vi "Decimator.vi"(4 "Size":u32=10, 6 "Mode":T1(ring)=enum."Non-sliding block", 8 "error in (no error)":errorcluster, 9 "Reset":bool, 10 "Enable":bool=TRUE, 11 "Signals":dynamicdata(graph)) -> (0 "error out":errorcluster, 1 "Data Valid":bool, 3 "Mean":dynamicdata(graph), 5 "Maximum":dynamicdata(graph))   [LabVIEW 2014]
doc: "Acquires a large number of data points and compresses the data points into a smaller number of points.\n--------------------\n\nThis Express VI is configured as follows:\n\nReduction Factor: 10\nReduction Method: Maximum\nReduction Method: Mean"
panel:
  in  "Tab Control":T2(tab)
  out "Sum":dynamicdata(graph)
  out "Median":dynamicdata(graph)
  out "Minimum":dynamicdata(graph)
  out "Last":dynamicdata(graph)
  out "Waveform Output":dynamicdata(graph)
  out "Signals In":dynamicdata(graph)
  in  "Functions":bool[](array[boolean])=[FALSE, TRUE, FALSE, TRUE, FALSE]
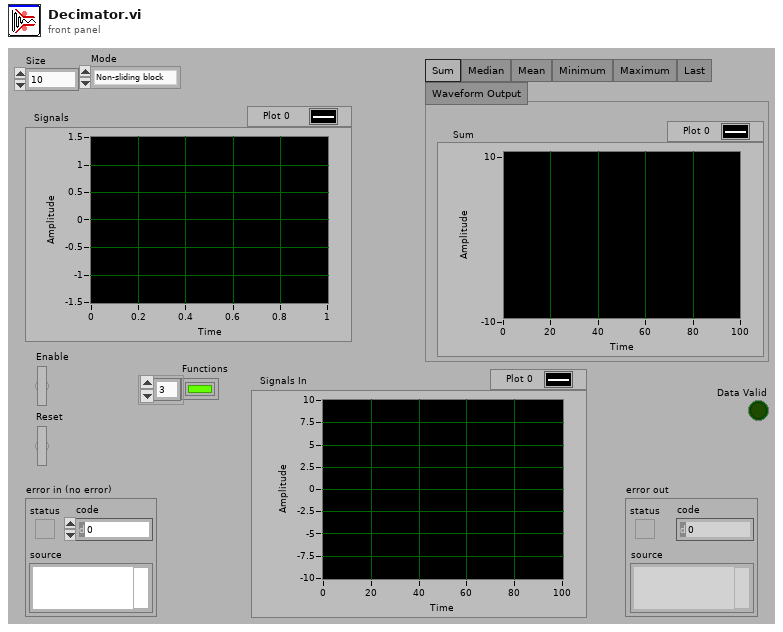
[diagram p1: front panel]
types:
  T1 = enum16{"Always", "Sliding Block", "Non-sliding block"}
  T2 = enum32{"Sum", "Median", "Mean", "Minimum", "Maximum", "Last", "Waveform Output"}
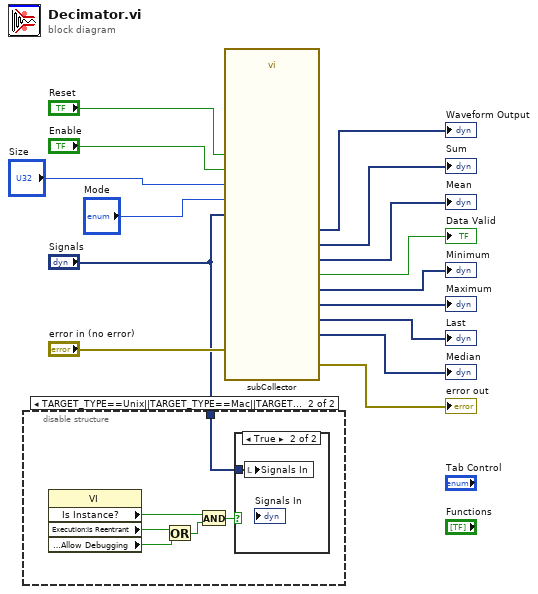
[diagram p0: block diagram]
diagram:
  n1 = disable-structure shown="TARGET_TYPE==Unix||TARGET_TYPE==Mac||TARGET_TYPE==Windows" {
    disable-tunnel: "Signals" -> [_ w16]
    frame condition #0 {
    }
    frame condition #1 (active) {
      n2 = property class="VI"() -> ("Is Instance?"=w20:bool, "Execution:Is Reentrant"=w18:bool, "Execution:Allow Debugging"=w17:bool)  [unwired: 2 in, 2 out]
      n3 = Or(x=w18, y=w17) -> (x .or. y?=w19:bool)
      n4 = And(x=w20, y=w19) -> (x .and. y?=w21:bool)
      n5 = case shown="True" w21 {
        tunnel: w16 -> [_ w22]
        frame False {
        }
        frame True {
          n6 = local write "Signals In"(w22) -> ()
        }
      }
    }
  }
  n7 = call <vilib>:"subCollector.vi"("Input"="Signals", "Reset"="Reset", "Enable"="Enable", "Mode"="Mode", "error in (no error)"="error in (no error)", "Size"="Size") -> ("Median"=→"Median":dynamicdata, "Min"=→"Minimum":dynamicdata, "Max"=→"Maximum":dynamicdata, "Last"=→"Last":dynamicdata, "Average"=→"Mean":dynamicdata, "Output Valid"=→"Data Valid":bool, "Waveform Output"=→"Waveform Output":dynamicdata, "Sum"=→"Sum":dynamicdata, "error out"=→"error out":errorcluster)  [unwired: 5 in]
